vi "Vector Addition.vi"(8 "error in (no error)":errorcluster) -> (0 "error out":errorcluster)   [LabVIEW 2023]
uses:
  <vilib>/addons/_JKI Toolkits/Caraya/classes/Assert/Assert True.vi
  <vilib>/addons/_JKI Toolkits/Caraya/classes/Test/Test.lvclass
  <vilib>/addons/_JKI Toolkits/Caraya/classes/Assert/Assert.lvclass
panel:
  # "Connector Pane"
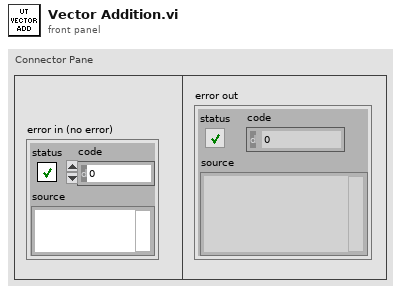
[diagram p1: front panel]
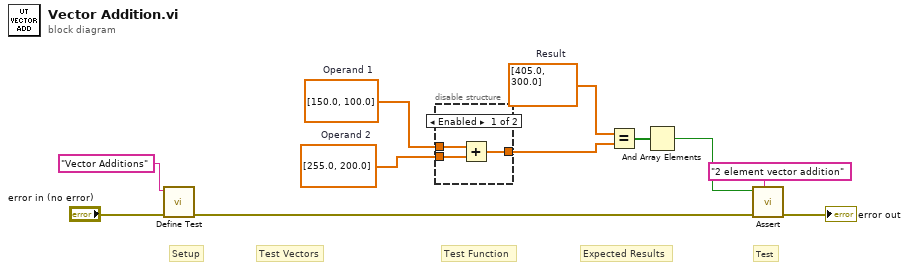
[diagram p0: block diagram]
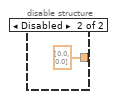
[diagram p2: hidden frame]
diagram:
  w3 = dbl[] [405.0, 300.0]  # Result
  w6 = dbl[] [255.0, 200.0]  # Operand 2
  w7 = dbl[] [150.0, 100.0]  # Operand 1
  # "Test Function"
  # "Expected Results"
  # "Test Vectors"
  # "Test"
  # "Setup"
  n1 = call <vilib>:"Define Test.vi"("error in (no error)"="error in (no error)", "Label (VI Title)"="Vector Additions") -> ("error out"=w8:errorcluster)  [unwired: 9 in]
  n2 = disable-structure shown="Enabled" {
    disable-tunnel: w7 -> [w14 _]
    disable-tunnel: w6 -> [w13 _]
    disable-tunnel: [w12 dbl[] [0.0, 0.0]] -> w5
    frame Enabled {
      n3 = Add(x=w14, y=w13) -> (x+y=w12:dbl[])
    }
    frame Disabled {
    }
  }
  n4 = Equal?(x=w3, y=w5) -> (x = y?=w4:bool[])
  n5 = And Array Elements(Boolean array=w4) -> (logical AND=w1:bool)
  n6 = call-poly <vilib>:"Assert.vi"("Label"="2 element vector addition" ("Label (VI Title)"), "error in (no error)"=w8, "True?"=w1) -> ("error out"=→"error out":errorcluster)  [unwired: 8 in]
